vi "3D_to_Screen.vi"(5 "X_3D":dbl, 9 "Y_3D":dbl) -> (6 "X":dbl, 10 "Y":dbl, 14 "Y_scaling":dbl)   [LabVIEW 2011]
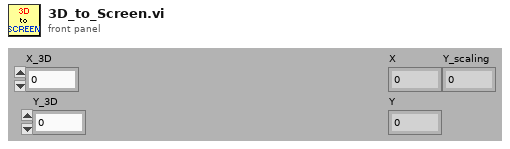
[diagram p1: front panel]
types:
  T1 = typedef "LVAllMonitorsDisplayTypeDef.ctl" = cluster{"Bounds":cluster{"Left":i16, "Top":i16, "Right":i16, "Bottom":i16}, "Depth":i16}[]
  T2 = cluster{"Bounds":cluster{"Left":i16, "Top":i16, "Right":i16, "Bottom":i16}, "Depth":i16}
  T3 = cluster{"Left":i16, "Top":i16, "Right":i16, "Bottom":i16}
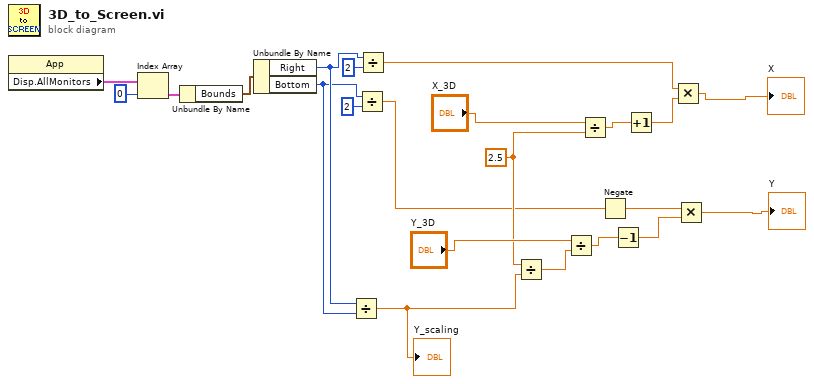
[diagram p0: block diagram]
diagram:
  w8 = 2.5 ("y")
  n1 = property class="App"() -> ("Disp.AllMonitors"=w19:T1)  [unwired: 2 in, 2 out]
  n2 = Index Array(array=w19, index=u16 0 ("Front Panel Window:Monitor")) -> (element=w21:T2)
  n3 = Unbundle By Name(w21) -> ("Bounds"=w18:T3)
  n4 = Unbundle By Name(w18) -> ("Right"=w11:i16, "Bottom"=w10:i16)
  n5 = Divide(x=w11, y=w10) -> (x/y=w5:dbl)
  "Y_scaling" <- w5
  n6 = Divide(x=w10, y=i16 2) -> (x/y=w7:dbl)
  n7 = Divide(x=w11, y=i16 2) -> (x/y=w15:dbl)
  n8 = Divide(x=w8, y=w5) -> (x/y=w9:dbl)
  n9 = Divide(x="Y_3D", y=w9) -> (x/y=w13:dbl)
  n10 = Divide(x="X_3D", y=w8) -> (x/y=w4:dbl)
  n11 = Negate(x=w7) -> (-x=w6:dbl)
  n12 = Decrement(x=w13) -> (x-1=w12:dbl)
  n13 = Increment(x=w4) -> (x+1=w3:dbl)
  n14 = Multiply(x=w15, y=w3) -> (x*y=→"X":dbl)
  n15 = Multiply(x=w6, y=w12) -> (x*y=→"Y":dbl)
